vi "DMC VIDoc Confluence.vi"(8 "Error in":errorcluster caption="Error in (no error)") -> ()   [LabVIEW 2023]
uses:
  Documentation Generation/TypeDefs/Git Type.ctl
  DMC CLI Confluence Documentation State.ctl
  <vilib>/Wiresmith Technology/G CLI/CLI Class/CLI.lvclass
  Documentation Generation/TypeDefs/File Change Map.ctl
  Confluence Settings.ctl
  Documentation Generation/Parsing/TypeDefs/Full Documentation Info.ctl
  Documentation Generation/Parsing/Project Documentation/Project Documentation.lvclass
  Documentation Generation/Parsing/Interface Documenation/Interface Documenation.lvclass
  Documentation Generation/Parsing/Class Documentation/Class Documentation.lvclass
  Documentation Generation/Parsing/Library Documentation/Library Documentation.lvclass
  Documentation Generation/Parsing/GUI Documentation/GUI Documentation.lvclass
  Documentation Generation/Parsing/LLB Documentation/LLB Documentation.lvclass
  <vilib>/Wiresmith Technology/G CLI/Argument Parser/Option Class/Option Configuration.ctl
  <vilib>/Wiresmith Technology/G CLI/Argument Parser/Option Class/Argument Type.ctl
  8042783b-93c0-44c7-9b89-4fb89b10c9de.vi
  g-CLI Interaction/g-CLI Interaction.lvclass
  C:/projects/DMC/GitHub/DMC CLI VIDoc/Source/Documentation Generation/UI Interaction/UI Interaction.lvclass
  Documentation Generation/Printers/Confluence Printer/VIDoc Printer - Confluence.lvclass
  <vilib>/Wiresmith Technology/G CLI/Argument Parser/Option Set Class/Option Set.lvclass
  <vilib>/Wiresmith Technology/G CLI/Argument Parser/Option Class/Option.lvclass
  Documentation Generation/Parsing/Documentation Parser/VIDoc Parser.lvclass
  Documentation Generation/Parsing/VIDoc Parsing.lvlib
panel:
  out "Confluence Token":string
  out "Confluence Email":string
  out "Confluence URL":string
  out "Use Data Center for Confluence Connection?":bool
  out "Use Login INI file for Confluence Connection?":bool
  out "Use Settings file for Confluence Connection Settings?":bool
  out "Top Page ID":string
  out "Source Paths":path[](array[path])
  out "Git Type":T1
  out "Run Git History?":bool
  out "Doc Settings Path":path
  out "Custom Parameters":string[](array[string])
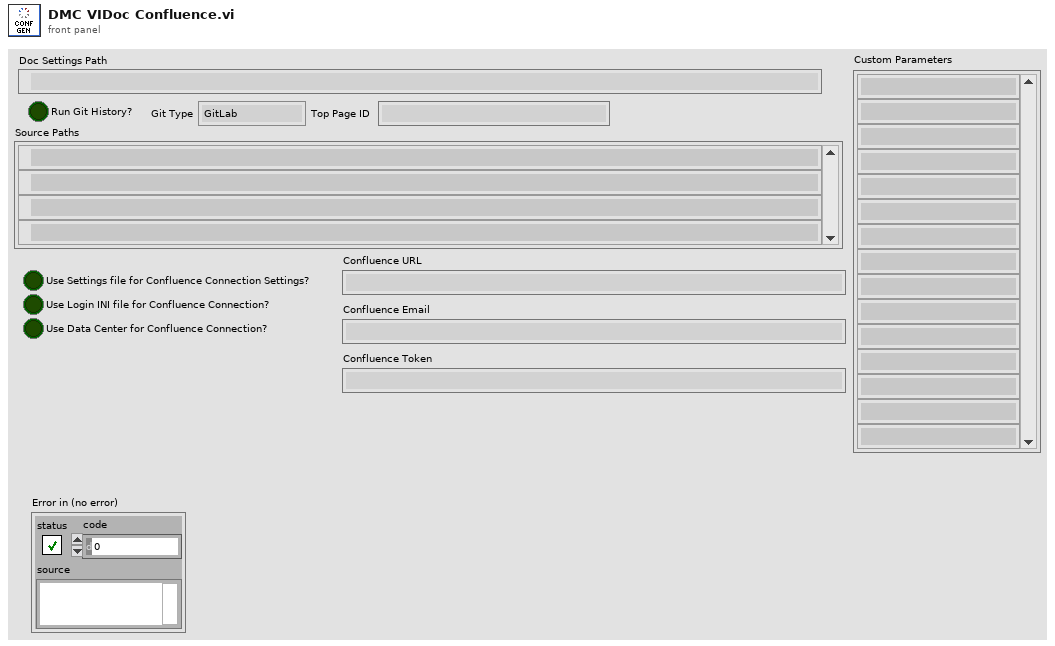
[diagram p1: front panel]
types:
  T1 = typedef "Git Type.ctl" = enum16{"GitLab", "GitHub", "BitBucket"}
  T2 = typedef "File Change Map.ctl" = map{string, cluster{"Timestamp":timestamp, "Commit Hash":string, "Author Name":string, "Branch":string, "Commit Hash URL":string}}
  T3 = typedef "Confluence Settings.ctl" = cluster{"Use INI?":bool, "URL":string, "Email":string, "Token":string, "Use Settings File?":bool, "Data Center?":bool}
  T4 = typedef "VIDoc Parsing.lvlib/Full Documentation Info.ctl" = cluster{"Projects":refnum<class "Project Documentation.lvclass">[], "Interfaces":refnum<class "Interface Documenation.lvclass">[], "Classes":refnum<class "Class Documentation.lvclass">[], "Libraries":refnum<class "Library Documentation.lvclass">[], "VI Members":refnum<class "GUI Documentation.lvclass">[], "Controls":refnum<class "GUI Documentation.lvclass">[], "LLBs":refnum<class "LLB Documentation.lvclass">[], "Bookmarked Map":map{string, refnum<class "GUI Documentation.lvclass">[]}}
  T5 = cluster{"CLI":refnum<class "CLI.lvclass">, "Working Directory":path, "Doc Settings Path":path, "Git History?":bool, "Git Type":T1, "File Change Map":T2, "Source Paths":path[], "Top Page ID":string, "Confluence Settings":T3, "Full Documentation":T4}
  T6 = typedef "DMC CLI Confluence Documentation State.ctl" = enum16{"Initialize", "Display Settings", "Git History", "Fetch Documentation", "Create Documentation", "Close", "Help"}
  T7 = enum16{"Doc Settings Path", "Git History", "Git Type", "Source Rel Paths", "Top Page ID", "Confluence Use Settings", "Confluence Use INI", "Confluence Type", "Confluence URL", "Confluence Email", "Confluence Token"}
  T8 = typedef "Option Parser.lvlib/Option.lvclass/Option Configuration.ctl" = cluster{"Option Type":T9, "Option Labels":string[], "Key":string, "Description":string, "Required":bool, "Default Value":string}
  T9 = typedef "Option Parser.lvlib/Option.lvclass/Argument Type.ctl" = enum16{"flag", "value"}
  T10 = enum16{"Doc Settings Path", "Git History", "Git Type", "Source Rel Paths", "Top Page ID", "Confluence Use Settings", "Confluence Use INI", "Confluence Type", "Confluence URL", "Confluence Email", "Confluence Token"}[]
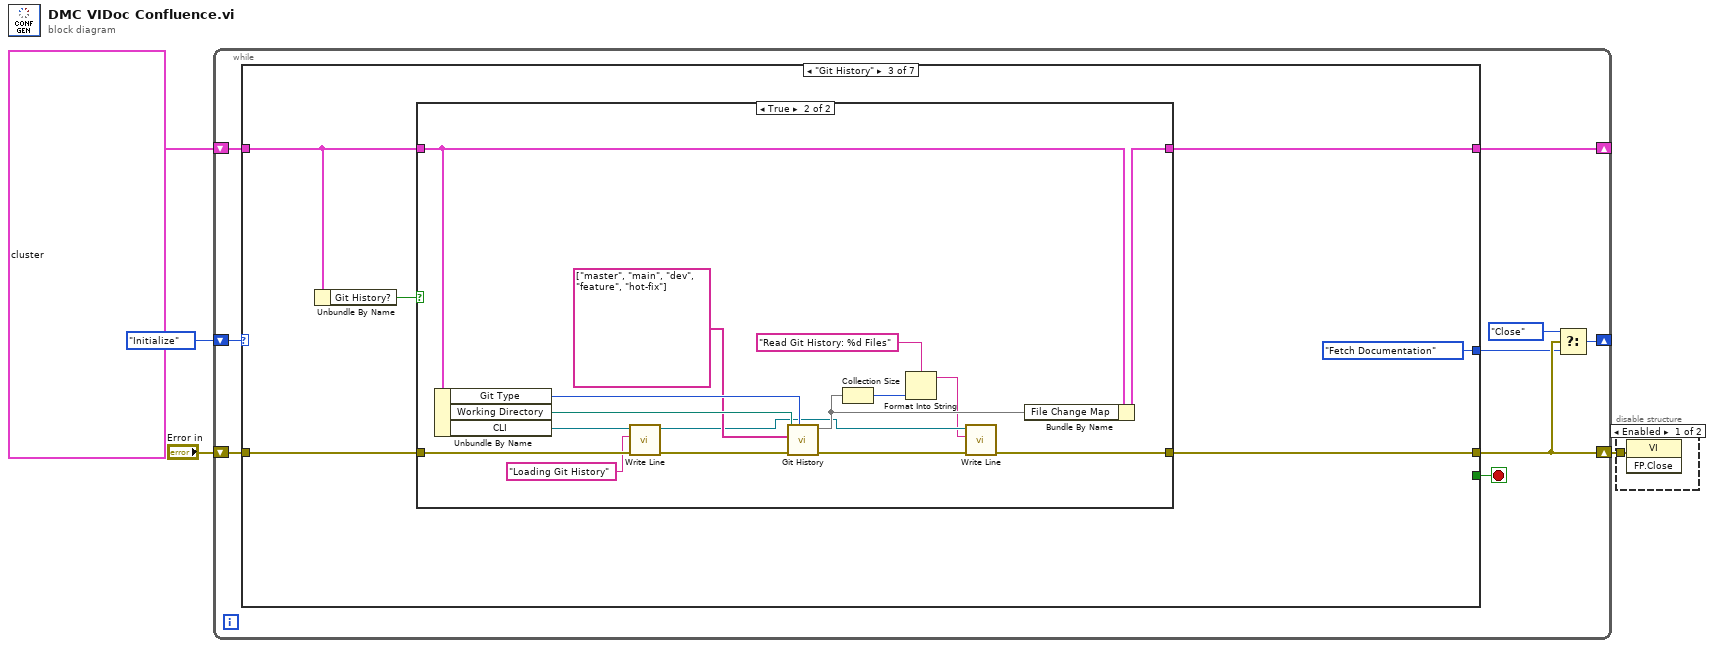
[diagram p0: block diagram]
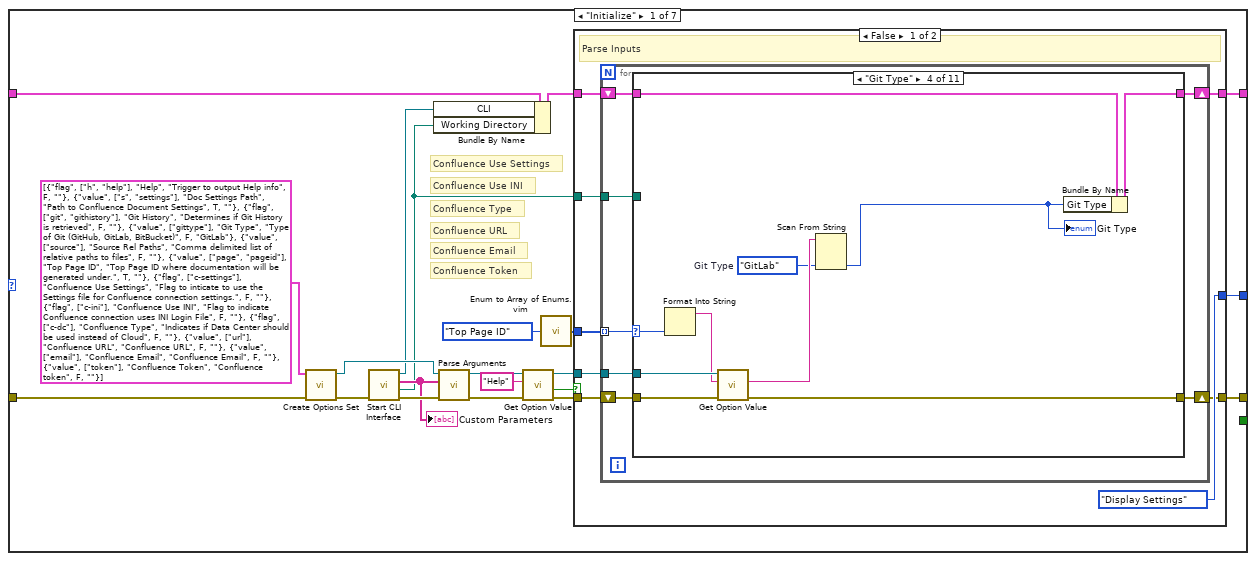
[diagram p3: hidden frame]
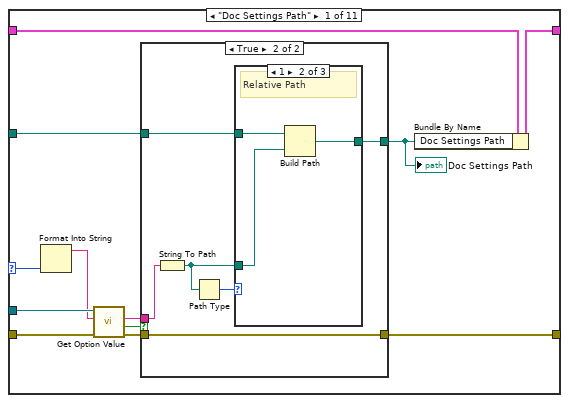
[diagram p4: hidden frame]
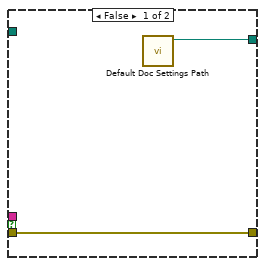
[diagram p5: hidden frame]
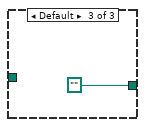
[diagram p7: hidden frame]
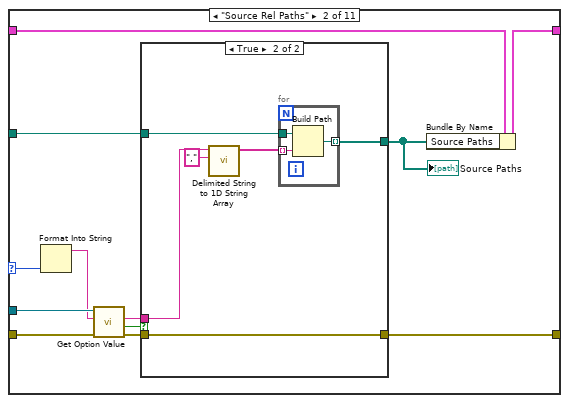
[diagram p8: hidden frame]
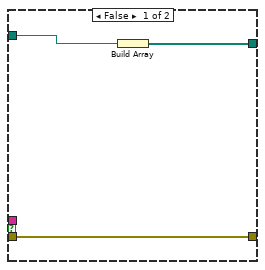
[diagram p9: hidden frame]
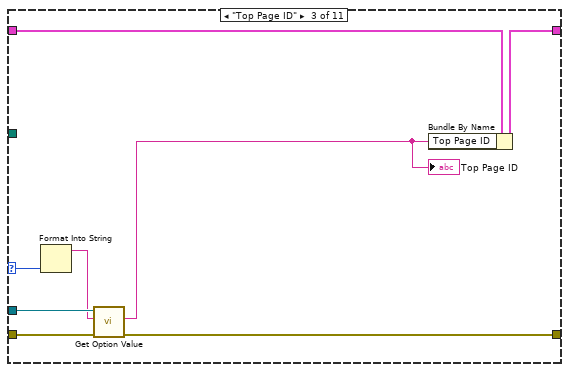
[diagram p10: hidden frame]
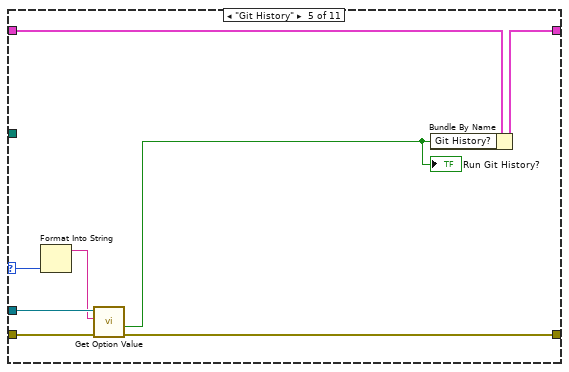
[diagram p11: hidden frame]
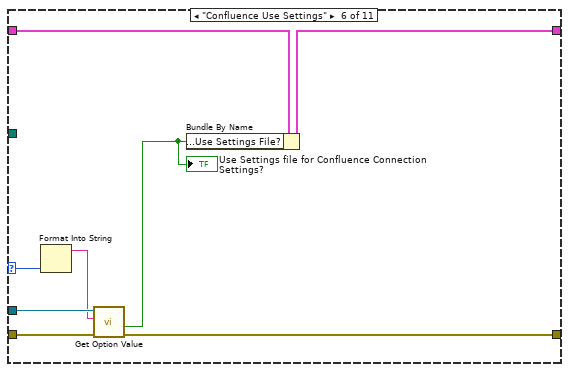
[diagram p12: hidden frame]
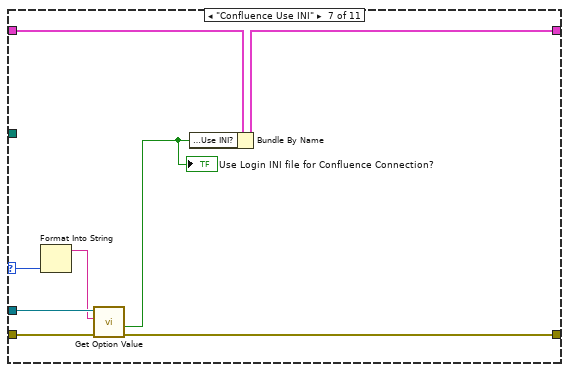
[diagram p13: hidden frame]
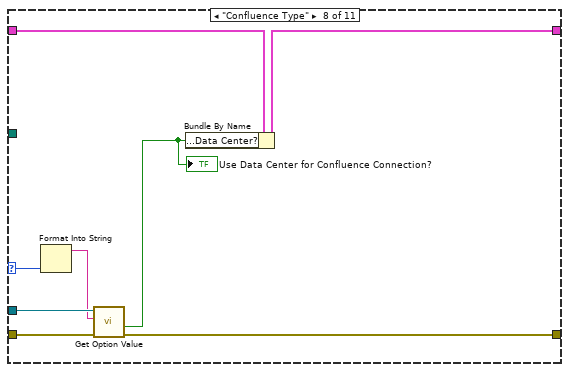
[diagram p14: hidden frame]
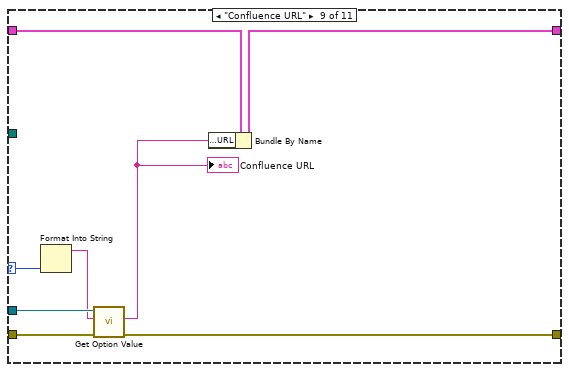
[diagram p15: hidden frame]
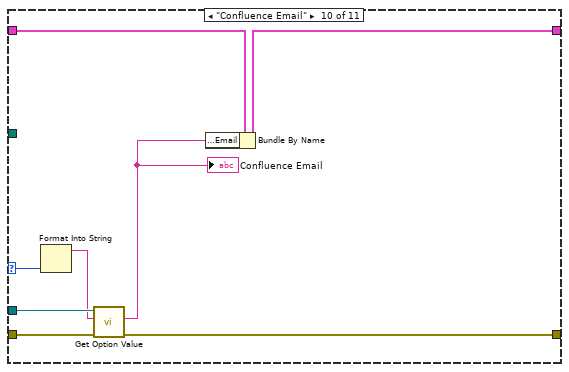
[diagram p16: hidden frame]
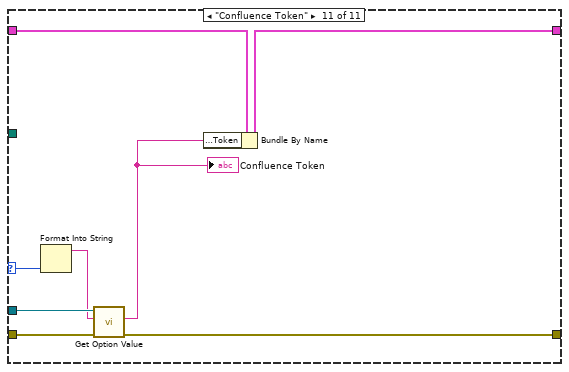
[diagram p17: hidden frame]
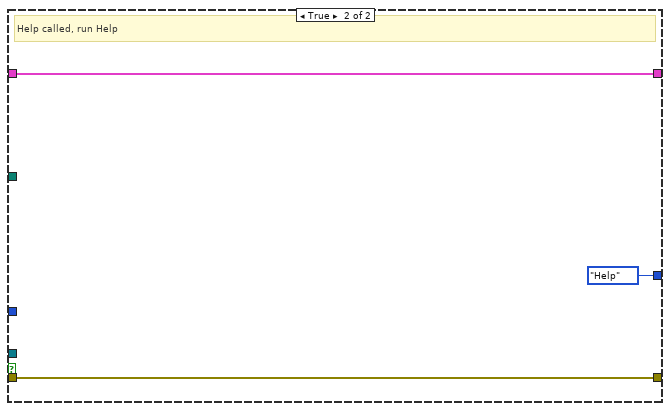
[diagram p18: hidden frame]
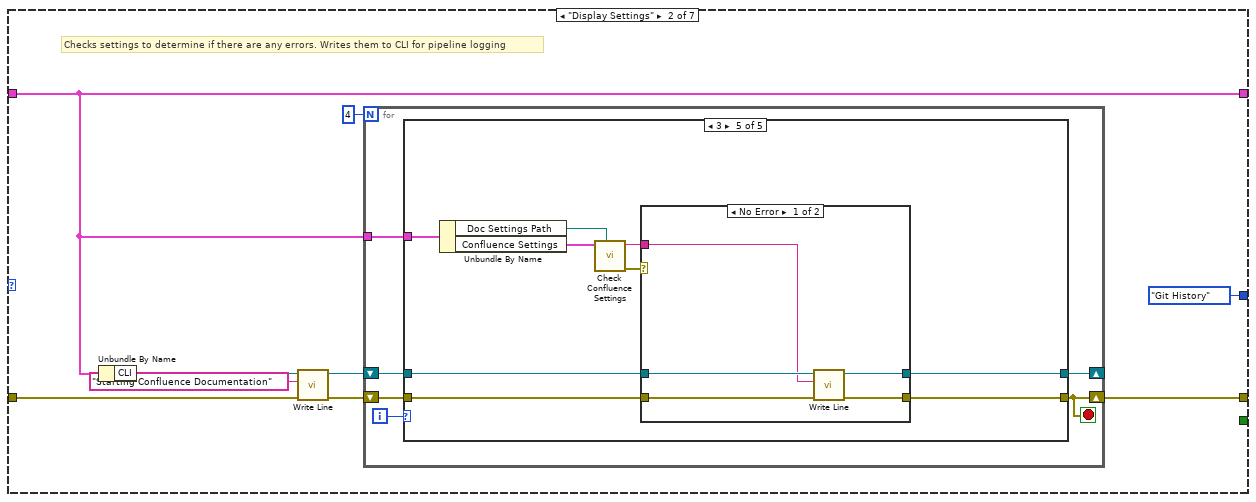
[diagram p19: hidden frame]
diagram:
  n1 = while {
    shift-right: [w8] -> _
    shift-left: DMC_CLI_Confluence_Documentation_State."Initialize" -> [w13]
    shift-right: [w10] -> w1
    shift-left: "Error in" -> [w12]
    shift-right: [w5] -> _
    shift-left: T5 {"CLI"=refnum, "Working Directory"=path "", "Doc Settings Path"=path "", "Git History?"=FALSE, "Git Type"=enum."GitLab", "File Change Map"={}, "Source Paths"=[], "Top Page ID"="", "Confluence Settings"={"Use INI?"=FALSE, "URL"="", "Email"="", "Token"="", "Use Settings File?"=FALSE, "Data Center?"=FALSE}, "Full Documentation"={"Projects"=[], "Interfaces"=[], "Classes"=[], "Libraries"=[], "VI Members"=[], "Controls"=[], "LLBs"=[], "Bookmarked Map"={}}} -> [w6]
    stop <- w7 stop-if-true
    n2 = case shown="\"Git History\"" w13 {
      tunnel: w12 -> [w26 w179 w264 w300 w314 w326 w336]
      tunnel: [w17 w184 w261 w284 w316 w327 w337] -> w10
      tunnel: [w19 DMC_CLI_Confluence_Documentation_State."Git History" DMC_CLI_Confluence_Documentation_State."Fetch Documentation" DMC_CLI_Confluence_Documentation_State."Create Documentation" DMC_CLI_Confluence_Documentation_State."Close" DMC_CLI_Confluence_Documentation_State."Close" DMC_CLI_Confluence_Documentation_State."Close"] -> w9
      tunnel: [_ _ _ _ _ TRUE _] -> w7
      tunnel: w6 -> [w25 w183 w262 w301 w315 w330 w334]
      tunnel: [w21 w183 w263 w295 w315 w330 w334] -> w5
      frame "Initialize" {
        # "Confluence Token"
        # "Confluence Email"
        # "Confluence URL"
        # "Confluence Type"
        # "Confluence Use INI"
        # "Confluence Use Settings"
        n3 = call <vilib>:"Create Options Set.vi"("error in (no error)"=w26, "Options"=T8[] [{"Option Type"=enum."flag", "Option Labels"=["h", "help"], "Key"="Help", "Description"="Trigger to output Help info", "Required"=FALSE, "Default Value"=""}, {"Option Type"=enum."value", "Option Labels"=["s", "settings"], "Key"="Doc Settings Path", "Description"="Path to Confluence Document Settings", "Required"=TRUE, "Default Value"=""}, {"Option Type"=enum."flag", "Option Labels"=["git", "githistory"], "Key"="Git History", "Description"="Determines if Git History is retrieved", "Required"=FALSE, "Default Value"=""}, {"Option Type"=enum."value", "Option Labels"=["gittype"], "Key"="Git Type", "Description"="Type of Git (GitHub, GitLab, BitBucket)", "Required"=FALSE, "Default Value"="GitLab"}, {"Option Type"=enum."value", "Option Labels"=["source"], "Key"="Source Rel Paths", "Description"="Comma delimited list of relative paths to files", "Required"=FALSE, "Default Value"=""}, {"Option Type"=enum."value", "Option Labels"=["page", "pageid"], "Key"="Top Page ID", "Description"="Top Page ID where documentation will be generated under.", "Required"=TRUE, "Default Value"=""}, {"Option Type"=enum."flag", "Option Labels"=["c-settings"], "Key"="Confluence Use Settings", "Description"="Flag to inticate to use the Settings file for Confluence connection settings.", "Required"=FALSE, "Default Value"=""}, {"Option Type"=enum."flag", "Option Labels"=["c-ini"], "Key"="Confluence Use INI", "Description"="Flag to indicate Confluence connection uses INI Login File", "Required"=FALSE, "Default Value"=""}, {"Option Type"=enum."flag", "Option Labels"=["c-dc"], "Key"="Confluence Type", "Description"="Indicates if Data Center should be used instead of Cloud", "Required"=FALSE, "Default Value"=""}, {"Option Type"=enum."value", "Option Labels"=["url"], "Key"="Confluence URL", "Description"="Confluence URL", "Required"=FALSE, "Default Value"=""}, {"Option Type"=enum."value", "Option Labels"=["email"], "Key"="Confluence Email", "Description"="Confluence Email", "Required"=FALSE, "Default Value"=""}, {"Option Type"=enum."value", "Option Labels"=["token"], "Key"="Confluence Token", "Description"="Confluence token", "Required"=FALSE, "Default Value"=""}]) -> ("error out"=w32:errorcluster, "Option Set out"=w31:refnum<class "Option Set.lvclass">)  [unwired: 8 in]
        n4 = call <vilib>:"Start CLI Interface.vi"("error in (no error)"=w32) -> ("error out"=w34:errorcluster, "Working Directory"=w14:path, "Custom Parameters"=w30:string[], "CLI out"=w24:refnum<class "CLI.lvclass">)  [unwired: 7 in]
        "Custom Parameters" <- w30
        n5 = Bundle By Name(cluster=w25, "CLI"=w24, "Working Directory"=w14) -> (w20:T5)
        n6 = call <vilib>:"Parse Arguments.vi"("error in (no error)"=w34, "Arguments"=w30, "Option Set in"=w31) -> ("error out"=w28:errorcluster, "Option Set out"=w27:refnum<class "Option Set.lvclass">)  [unwired: 5 in, 2 out]
        n7 = call <vilib>:"Get Option Value.vi"("error in (no error)"=w28, "Option Key"="Help", "Option Set in"=w27) -> ("error out"=w18:errorcluster, "Set"=w23:bool, "Option Set out"=w22:refnum<class "Option Set.lvclass">)  [unwired: 5 in, 1 out]
        n8 = call "Enum to Array of Enums.vim"("enum"=T7."Top Page ID") -> ("array of enums"=w15:T10)
        n9 = case shown="False" w23 {
          tunnel: w22 -> [w41 _]
          tunnel: [w39 w175] -> w21
          tunnel: w20 -> [w40 w175]
          tunnel: [DMC_CLI_Confluence_Documentation_State."Display Settings" DMC_CLI_Confluence_Documentation_State."Help"] -> w19
          tunnel: w18 -> [w42 w173]
          tunnel: [w35 w173] -> w17
          tunnel: w15 -> [w38 _]
          tunnel: w14 -> [w37 _]
          frame False {
            # "Parse Inputs"
            n10 = for {
              shift-right: [w44] -> w35
              shift-left: w42 -> [w45]
              tunnel: w41 -> [w46]
              shift-right: [w47] -> w39
              shift-left: w40 -> [w48]
              tunnel: w38 -> [w49] mode=indexing
              tunnel: w37 -> [w43]
              n11 = case shown="\"Git Type\"" w49 {
                selector: w49 -> [w58 w83 w103 w113 w121 w129 w137 w145 w153 w161 w169]
                tunnel: w48 -> [w61 w86 w106 w116 w124 w132 w140 w148 w156 w164 w172]
                tunnel: [w52 w77 w100 w111 w118 w126 w134 w142 w150 w158 w166] -> w47
                tunnel: w46 -> [w59 w84 w104 w114 w122 w130 w138 w146 w154 w162 w170]
                tunnel: w45 -> [w60 w85 w105 w115 w123 w131 w139 w147 w155 w163 w171]
                tunnel: [w53 w78 w101 w107 w119 w127 w135 w143 w151 w159 w167] -> w44
                tunnel: w43 -> [w50 w75 _ _ _ _ _ _ _ _ _]
                frame "Doc Settings Path" {
                  n12 = Format Into String(w58) -> (resulting string=w57:string)  [unwired: 3 in, 1 out]
                  n13 = call <vilib>:"Get Option Value.vi"("error in (no error)"=w60, "Option Key"=w57, "Option Set in"=w59) -> ("error out"=w56:errorcluster, "Set"=w54:bool, "Value"=w55:string)  [unwired: 5 in, 1 out]
                  n14 = case shown="True" w54 {
                    tunnel: w56 -> [w62 w69]
                    tunnel: w55 -> [_ w68]
                    tunnel: [w62 w69] -> w53
                    tunnel: [w63 w65] -> w51
                    tunnel: w50 -> [_ w64]
                    frame False {
                      n15 = call "Default Doc Settings Path.vi"() -> ("Default Doc Settings Path"=w63:path)  [unwired: 11 in]
                    }
                    frame True {
                      n16 = String To Path(string=w68) -> (path=w66:path)
                      n17 = Path Type(1:w66) -> (0:w67:i16)
                      n18 = case shown="1" w67 {
                        tunnel: w66 -> [w70 w72 _]
                        tunnel: [w70 w71 path ""] -> w65
                        tunnel: w64 -> [_ w73 _]
                        frame 0 {
                          # "Absolute Path"
                        }
                        frame 1 {
                          # "Relative Path"
                          n19 = Build Path(base path=w73, name or relative path=w72) -> (appended path=w71:path)
                        }
                        frame Default {
                        }
                      }
                    }
                  }
                  "Doc Settings Path" <- w51
                  n20 = Bundle By Name(cluster=w61, "Doc Settings Path"=w51) -> (w52:T5)
                }
                frame "Source Rel Paths" {
                  n21 = Format Into String(w83) -> (resulting string=w82:string)  [unwired: 3 in, 1 out]
                  n22 = call <vilib>:"Get Option Value.vi"("error in (no error)"=w85, "Option Key"=w82, "Option Set in"=w84) -> ("error out"=w81:errorcluster, "Set"=w79:bool, "Value"=w80:string)  [unwired: 5 in, 1 out]
                  n23 = case shown="True" w79 {
                    tunnel: w81 -> [w89 w95]
                    tunnel: w80 -> [_ w94]
                    tunnel: [w89 w95] -> w78
                    tunnel: [w87 w92] -> w76
                    tunnel: w75 -> [w88 w91]
                    frame False {
                      n24 = Build Array(w88) -> (w87:path[])
                    }
                    frame True {
                      n25 = call <vilib>:"Delimited String to 1D String Array.vi"("delimiter"=",", "delimited string"=w94) -> ("string array"=w90:string[])  [unwired: 9 in]
                      n26 = for {
                        tunnel: w91 -> [w98]
                        tunnel: w90 -> [w97] mode=indexing
                        tunnel: [w96] -> w92 mode=indexing
                        n27 = Build Path(base path=w98, name or relative path=w97) -> (appended path=w96:path)
                      }
                    }
                  }
                  "Source Paths" <- w76
                  n28 = Bundle By Name(cluster=w86, "Source Paths"=w76) -> (w77:T5)
                }
                frame "Top Page ID" {
                  n29 = Format Into String(w103) -> (resulting string=w102:string)  [unwired: 3 in, 1 out]
                  n30 = call <vilib>:"Get Option Value.vi"("error in (no error)"=w105, "Option Key"=w102, "Option Set in"=w104) -> ("error out"=w101:errorcluster, "Value"=w99:string)  [unwired: 5 in, 2 out]
                  "Top Page ID" <- w99
                  n31 = Bundle By Name(cluster=w106, "Top Page ID"=w99) -> (w100:T5)
                }
                frame "Git Type" {
                  w109 = Git_Type."GitLab"  # Git Type
                  n32 = Format Into String(w113) -> (resulting string=w112:string)  [unwired: 3 in, 1 out]
                  n33 = call <vilib>:"Get Option Value.vi"("error in (no error)"=w115, "Option Key"=w112, "Option Set in"=w114) -> ("error out"=w107:errorcluster, "Value"=w110:string)  [unwired: 5 in, 2 out]
                  n34 = Scan From String(input string=w110, default 1=w109) -> (output 1=w108:T1)  [unwired: 3 in, 3 out]
                  "Git Type" <- w108
                  n35 = Bundle By Name(cluster=w116, "Git Type"=w108) -> (w111:T5)
                }
                frame "Git History" {
                  n36 = Format Into String(w121) -> (resulting string=w120:string)  [unwired: 3 in, 1 out]
                  n37 = call <vilib>:"Get Option Value.vi"("error in (no error)"=w123, "Option Key"=w120, "Option Set in"=w122) -> ("error out"=w119:errorcluster, "Set"=w117:bool)  [unwired: 5 in, 2 out]
                  "Run Git History?" <- w117
                  n38 = Bundle By Name(cluster=w124, "Git History?"=w117) -> (w118:T5)
                }
                frame "Confluence Use Settings" {
                  n39 = Format Into String(w129) -> (resulting string=w128:string)  [unwired: 3 in, 1 out]
                  n40 = call <vilib>:"Get Option Value.vi"("error in (no error)"=w131, "Option Key"=w128, "Option Set in"=w130) -> ("error out"=w127:errorcluster, "Set"=w125:bool)  [unwired: 5 in, 2 out]
                  "Use Settings file for Confluence Connection Settings?" <- w125
                  n41 = Bundle By Name(cluster=w132, "Confluence Settings.Use Settings File?"=w125) -> (w126:T5)
                }
                frame "Confluence Use INI" {
                  n42 = Format Into String(w137) -> (resulting string=w136:string)  [unwired: 3 in, 1 out]
                  n43 = call <vilib>:"Get Option Value.vi"("error in (no error)"=w139, "Option Key"=w136, "Option Set in"=w138) -> ("error out"=w135:errorcluster, "Set"=w133:bool)  [unwired: 5 in, 2 out]
                  "Use Login INI file for Confluence Connection?" <- w133
                  n44 = Bundle By Name(cluster=w140, "Confluence Settings.Use INI?"=w133) -> (w134:T5)
                }
                frame "Confluence Type" {
                  n45 = Format Into String(w145) -> (resulting string=w144:string)  [unwired: 3 in, 1 out]
                  n46 = call <vilib>:"Get Option Value.vi"("error in (no error)"=w147, "Option Key"=w144, "Option Set in"=w146) -> ("error out"=w143:errorcluster, "Set"=w141:bool)  [unwired: 5 in, 2 out]
                  "Use Data Center for Confluence Connection?" <- w141
                  n47 = Bundle By Name(cluster=w148, "Confluence Settings.Data Center?"=w141) -> (w142:T5)
                }
                frame "Confluence URL" {
                  n48 = Format Into String(w153) -> (resulting string=w152:string)  [unwired: 3 in, 1 out]
                  n49 = call <vilib>:"Get Option Value.vi"("error in (no error)"=w155, "Option Key"=w152, "Option Set in"=w154) -> ("error out"=w151:errorcluster, "Value"=w149:string)  [unwired: 5 in, 2 out]
                  "Confluence URL" <- w149
                  n50 = Bundle By Name(cluster=w156, "Confluence Settings.URL"=w149) -> (w150:T5)
                }
                frame "Confluence Email" {
                  n51 = Format Into String(w161) -> (resulting string=w160:string)  [unwired: 3 in, 1 out]
                  n52 = call <vilib>:"Get Option Value.vi"("error in (no error)"=w163, "Option Key"=w160, "Option Set in"=w162) -> ("error out"=w159:errorcluster, "Value"=w157:string)  [unwired: 5 in, 2 out]
                  "Confluence Email" <- w157
                  n53 = Bundle By Name(cluster=w164, "Confluence Settings.Email"=w157) -> (w158:T5)
                }
                frame "Confluence Token" {
                  n54 = Format Into String(w169) -> (resulting string=w168:string)  [unwired: 3 in, 1 out]
                  n55 = call <vilib>:"Get Option Value.vi"("error in (no error)"=w171, "Option Key"=w168, "Option Set in"=w170) -> ("error out"=w167:errorcluster, "Value"=w165:string)  [unwired: 5 in, 2 out]
                  "Confluence Token" <- w165
                  n56 = Bundle By Name(cluster=w172, "Confluence Settings.Token"=w165) -> (w166:T5)
                }
              }
            }
          }
          frame True {
            # "Help called, run Help"
          }
        }
      }
      frame "Display Settings" {
        # "Checks settings to determine if there are any errors. Writes them to CLI for pipeline logging"
        n57 = Unbundle By Name(w183) -> ("CLI"=w180:refnum<class "CLI.lvclass">)
        n58 = call <vilib>:"Write Line.vi"("error in (no error)"=w179, "Text to Write"="Starting Confluence Documentation", "CLI in"=w180) -> ("error out"=w178:errorcluster, "CLI out"=w177:refnum<class "CLI.lvclass">)  [unwired: 7 in]
        n59 = for {
          N: 4 -> [_]
          shift-right: [w185] -> w184
          shift-left: w178 -> [w189]
          shift-right: [w188] -> _
          shift-left: w177 -> [w190]
          tunnel: w183 -> [w186]
          i -> [w187]
          stop <- w185 stop-if-true
          n60 = case shown="3" w187 {
            tunnel: w190 -> [w191 w199 w224 w231 w248]
            tunnel: [w192 w198 w223 w230 w247] -> w185
            tunnel: w189 -> [w192 w197 w222 w229 w249]
            tunnel: [w191 w196 w221 w228 w246] -> w188
            tunnel: w186 -> [_ w195 w220 w227 w252]
            frame Default {
            }
            frame 0 {
              n61 = Unbundle By Name(w195) -> ("Doc Settings Path"=w194:path)
              n62 = call "File Exists.vi"("Path"=w194) -> ("Exists?"=w193:bool)  [unwired: 9 in, 1 out]
              n63 = case shown="True" w193 {
                tunnel: w199 -> [w206 w213]
                tunnel: [w204 w212] -> w198
                tunnel: w197 -> [w205 w211]
                tunnel: [w206 w210] -> w196
                tunnel: w194 -> [w201 w208]
                frame False {
                  n64 = Format Into String(format string="Documentation Settings File Doesn't Exist: %s", w201) -> (resulting string=w200:string)  [unwired: 2 in, 1 out]
                  n65 = call <vilib>:"Error Cluster From Error Code.vi"("error in (no error)"=w205, "error message (\"\")"=w200, "error code (0)"=5555) -> ("error out"=w204:errorcluster)  [unwired: 6 in]
                }
                frame True {
                  n66 = Format Into String(format string="Documentation Settings Path: %s", w208) -> (resulting string=w207:string)  [unwired: 2 in, 1 out]
                  n67 = call <vilib>:"Write Line.vi"("error in (no error)"=w211, "Text to Write"=w207, "CLI in"=w213) -> ("error out"=w212:errorcluster, "CLI out"=w210:refnum<class "CLI.lvclass">)  [unwired: 7 in]
                }
              }
            }
            frame 1 {
              n68 = Unbundle By Name(w220) -> ("Source Paths"=w217:path[])
              n69 = Path To String(path=w217) -> (string=w216:string[])
              n70 = call <vilib>:"1D String Array to Delimited String.vi"("delimiter"="\r\n", "string array"=w216) -> ("delimited string"=w214:string)  [unwired: 9 in]
              n71 = Format Into String(format string="Source Paths: %s", w214) -> (resulting string=w218:string)  [unwired: 2 in, 1 out]
              n72 = call <vilib>:"Write Line.vi"("error in (no error)"=w222, "Text to Write"=w218, "CLI in"=w224) -> ("error out"=w223:errorcluster, "CLI out"=w221:refnum<class "CLI.lvclass">)  [unwired: 7 in]
            }
            frame 2 {
              n73 = Unbundle By Name(w227) -> ("Top Page ID"=w226:string)
              n74 = Empty String/Path?(string/path=w226) -> (empty?=w225:bool)
              n75 = case shown="False" w225 {
                tunnel: w231 -> [w238 w243]
                tunnel: [w237 w241] -> w230
                tunnel: w229 -> [w236 w242]
                tunnel: [w235 w243] -> w228
                tunnel: w226 -> [w232 _]
                frame False {
                  n76 = Format Into String(format string="Top Page ID: %s", w232) -> (resulting string=w233:string)  [unwired: 2 in, 1 out]
                  n77 = call <vilib>:"Write Line.vi"("error in (no error)"=w236, "Text to Write"=w233, "CLI in"=w238) -> ("error out"=w237:errorcluster, "CLI out"=w235:refnum<class "CLI.lvclass">)  [unwired: 7 in]
                }
                frame True {
                  n78 = call <vilib>:"Error Cluster From Error Code.vi"("error in (no error)"=w242, "error message (\"\")"="No Top Page ID Assigned." ("error message (\"\")"), "error code (0)"=5556) -> ("error out"=w241:errorcluster)  [unwired: 6 in]
                }
              }
            }
            frame 3 {
              n79 = Unbundle By Name(w252) -> ("Doc Settings Path"=w251:path, "Confluence Settings"=w250:T3)
              n80 = call "Check Confluence Settings.vi"("Settings Path"=w251, "Confluence Settings"=w250) -> ("Error out"=w244:errorcluster, "String"=w245:string)  [unwired: 8 in]
              n81 = case shown="No Error" w244 {
                selector: w244 -> [_ w259]
                tunnel: w249 -> [w257 _]
                tunnel: w248 -> [w256 w258]
                tunnel: [w255 w259] -> w247
                tunnel: [w254 w258] -> w246
                tunnel: w245 -> [w253 _]
                frame No Error {
                  n82 = call <vilib>:"Write Line.vi"("error in (no error)"=w257, "Text to Write"=w253, "CLI in"=w256) -> ("error out"=w255:errorcluster, "CLI out"=w254:refnum<class "CLI.lvclass">)  [unwired: 7 in]
                }
                frame Error {
                }
              }
            }
          }
        }
      }
      frame "Git History" {
        n83 = Unbundle By Name(w262) -> ("Git History?"=w265:bool)
        n84 = case shown="True" w265 {
          tunnel: w264 -> [w267 w283]
          tunnel: [w266 w275] -> w263
          tunnel: w262 -> [w266 w276]
          tunnel: [w267 w272] -> w261
          frame False {
          }
          frame True {
            n85 = Unbundle By Name(w276) -> ("Git Type"=w278:T1, "Working Directory"=w279:path, "CLI"=w282:refnum<class "CLI.lvclass">)
            n86 = call <vilib>:"Write Line.vi"("error in (no error)"=w283, "Text to Write"="Loading Git History", "CLI in"=w282) -> ("error out"=w280:errorcluster, "CLI out"=w271:refnum<class "CLI.lvclass">)  [unwired: 7 in]
            n87 = call "Git History.vi"("Git Type"=w278, "Error in"=w280, "Branch Hierarchy"=string[] ["master", "main", "dev", "feature", "hot-fix"], "Working Directory"=w279) -> ("Error out"=w273:errorcluster, "File Change Map"=w274:T2)  [unwired: 6 in]
            n88 = Collection Size(1:w274) -> (0:w269:i32)
            n89 = Format Into String(format string="Read Git History: %d Files", w269) -> (resulting string=w268:string)  [unwired: 2 in, 1 out]
            n90 = call <vilib>:"Write Line.vi"("error in (no error)"=w273, "Text to Write"=w268, "CLI in"=w271) -> ("error out"=w272:errorcluster)  [unwired: 7 in, 1 out]
            n91 = Bundle By Name(cluster=w276, "File Change Map"=w274) -> (w275:T5)
          }
        }
      }
      frame "Fetch Documentation" {
        n92 = Unbundle By Name(w301) -> ("Source Paths"=w288:path[], "Doc Settings Path"=w291:path, "CLI"=w299:refnum<class "CLI.lvclass">)
        n93 = call <vilib>:"Write Line.vi"("error in (no error)"=w300, "Text to Write"="Parsing Source Files", "CLI in"=w299) -> ("error out"=w297:errorcluster, "CLI out"=w296:refnum<class "CLI.lvclass">)  [unwired: 7 in]
        n94 = call "Wrap g-CLI.vi"("error in (no error)"=w297, "CLI"=w296) -> ("error out"=w292:errorcluster, "g-CLI Interaction out"=w293:refnum<class "g-CLI Interaction.lvclass">)  [unwired: 8 in]
        n95 = call "Initialize.vi"("error in (no error)"=w292, "Settings Path"=w291, "UI Interaction"=w293) -> ("error out"=w289:errorcluster, "VIDoc Parser Out"=w290:refnum<class "VIDoc Parser.lvclass">)  [unwired: 7 in]
        n96 = call "Fetch Full Documentation.vi"("error in (no error)"=w289, "File Paths"=w288, "VIDoc Parser In"=w290) -> ("error out"=w286:errorcluster, "Full Documentation"=w287:T4, "VIDoc Parser Out"=w285:refnum<class "VIDoc Parser.lvclass">)  [unwired: 6 in]
        n97 = call "Close.vi"("error in (no error)"=w286, "VIDoc Parser In"=w285) -> ("error out"=w284:errorcluster)  [unwired: 9 in]
        n98 = Bundle By Name(cluster=w301, "Full Documentation"=w287) -> (w295:T5)
      }
      frame "Create Documentation" {
        n99 = Unbundle By Name(w315) -> ("Full Documentation"=w311:T4, "Doc Settings Path"=w312:path, "Top Page ID"=w307:string, "Working Directory"=w308:path, "File Change Map"=w309:T2, "Confluence Settings"=w303:T3, "CLI"=w302:refnum<class "CLI.lvclass">)
        n100 = call "Wrap g-CLI.vi"("error in (no error)"=w314, "CLI"=w302) -> ("error out"=w306:errorcluster, "g-CLI Interaction out"=w313:refnum<class "g-CLI Interaction.lvclass">)  [unwired: 8 in]
        n101 = call "Determine Confluence Connection.vi"("Error in"=w306, "Confluence Settings"=w303) -> ("Error out"=w305:errorcluster, "Confluence"=w304:refnum<class "Confluence.lvclass">)  [unwired: 8 in]
        n102 = call "Construct.vi"("File Change Map"=w309, "error in (no error)"=w305, "Working Directory"=w308, "Top Page ID"=w307, "Confluence"=w304) -> ("error out"=w323:errorcluster, "VIDoc Printer - Confluence Out"=w324:refnum<class "VIDoc Printer - Confluence.lvclass">)  [unwired: 5 in]
        n103 = call-dynamic "Initialize.vi"("UI Interaction"=w313, "error in (no error)"=w323, "Settings Path"=w312, "VIDoc Printer - Confluence In"=w324) -> ("error out"=w321:errorcluster, "VIDoc Printer - Confluence Out"=w322:refnum<class "VIDoc Printer - Confluence.lvclass">)  [unwired: 6 in]
        n104 = call-dynamic "Report.vi"("error in (no error)"=w321, "Full Documentation"=w311, "VIDoc Printer In"=w322) -> ("error out"=w319:errorcluster, "VIDoc Printer Out"=w320:refnum<class "VIDoc Printer - Confluence.lvclass">)  [unwired: 7 in]
        n105 = call "Publish Pages.vi"("error in (no error)"=w319, "VIDoc Printer - Confluence In"=w320) -> ("error out"=w317:errorcluster, "VIDoc Printer - Confluence Out"=w318:refnum<class "VIDoc Printer - Confluence.lvclass">)  [unwired: 8 in]
        n106 = call-dynamic "Close.vi"("error in (no error)"=w317, "VIDoc Printer - Confluence In"=w318) -> ("error out"=w316:errorcluster)  [unwired: 9 in]
      }
      frame "Close" {
        n107 = Unbundle By Name(w330) -> ("CLI"=w328:refnum<class "CLI.lvclass">)
        n108 = call <vilib>:"Write Line.vi"("Text to Write"="Exiting Confluence Documentation", "CLI in"=w328) -> ("CLI out"=w325:refnum<class "CLI.lvclass">)  [unwired: 8 in, 1 out]
        n109 = call <vilib>:"Exit With Error Cluster Code.vi"("error in (no error)"=w326, "CLI in"=w325) -> ("error out"=w327:errorcluster)  [unwired: 9 in]
      }
      frame "Help" {
        n110 = Unbundle By Name(w334) -> ("CLI"=w333:refnum<class "CLI.lvclass">)
        n111 = call <vilib>:"Write Line.vi"("error in (no error)"=w336, "Text to Write"="-------required arguments-------\n-settings <absolute or relative to working directory relative path to Doc Settings file. defaults to Default.json included with app>\n-pageid <Page ID for the top level Confluence Page that documentation will be generated under>\n\n-------optional arguments-------\n-git <Flag to include Git History in the documentation>\n-gittype <Indicates which Git repo type the Git History would check. Defaults to GitLab, also allows GitHub and BitBucket>\n-source <comma seperated string of all relative file paths within working directory to include. Recursive search. Defaults to whole working directory>\n-c-settings <Flag to indicate use the Confluence connection settings from within the Doc Settings File>\n-c-ini <Flag to indicate using the Login INI file for Confluence connections>\n-c-dc <Indicates Confluence type. If flag present then uses Data Center, otherwise uses Cloud>\n-url <Confluence URL>\n-email <Confluence Email>\n-token <Confluence Access Token>\n-help <Returns this help information>" ("string"), "CLI in"=w333) -> ("error out"=w337:errorcluster)  [unwired: 7 in, 1 out]
      }
    }
    n112 = Select(t=DMC_CLI_Confluence_Documentation_State."Close", s=w10, f=w9) -> (s? t:f=w8:T6)
  }
  n113 = disable-structure shown="Enabled" {
    disable-tunnel: w1 -> [w339 _]
    frame Enabled {
      n114 = invoke class="VI" method="FP.Close"(error in=w339) -> ()  [unwired: 2 in, 3 out]
    }
    frame Disabled {
    }
  }
